vi "hw1-2.vi"() -> ()   [LabVIEW 2014]
panel:
  in  "Length of line 1":dbl
  in  "stop":bool
  out "2D Picture":picture
  in  "Angle 2":dbl(slide) scale=0.0..360.0
  in  "Length of line 2":dbl
  in  "Angle 1":dbl(slide) scale=0.0..360.0
  out "Line 1End y":dbl
  out "Line 1End x":dbl
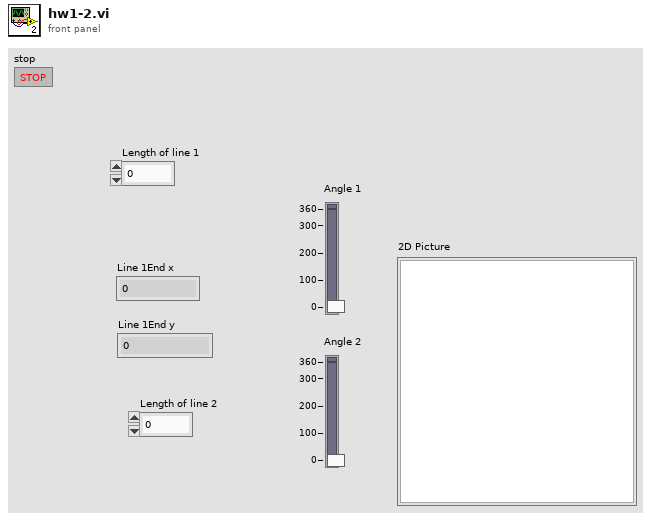
[diagram p1: front panel]
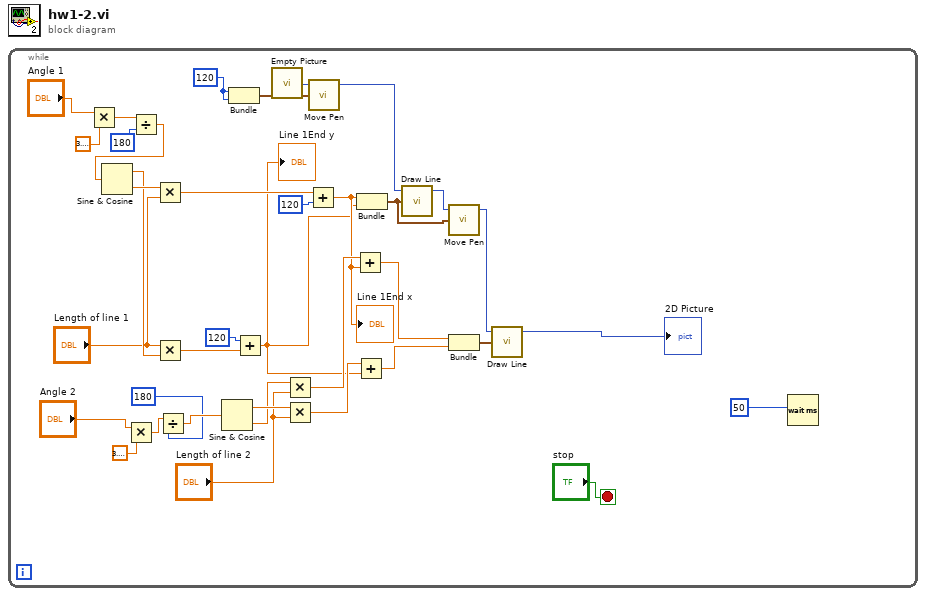
[diagram p0: block diagram]
diagram:
  n1 = while {
    stop <- "stop" stop-if-true
    w27 = 120
    n2 = Multiply(x="Angle 1", y=3.141592653589793) -> (x*y=w6:dbl)
    n3 = Multiply(x="Angle 2", y=3.141592653589793) -> (x*y=w2:dbl)
    n4 = Divide(x=w6, y=180) -> (x/y=w5:dbl)
    n5 = Sine & Cosine(0:w5) -> (1:w35:dbl, 2:w37:dbl)
    n6 = Multiply(x=w37, y="Length of line 1") -> (x*y=w36:dbl)
    n7 = Multiply(x="Length of line 1", y=w35) -> (x*y=w34:dbl)
    n8 = Divide(x=w2, y=180) -> (x/y=w3:dbl)
    n9 = Sine & Cosine(0:w3) -> (1:w33:dbl, 2:w32:dbl)
    n10 = Bundle(w27, w27) -> (w26:cluster{i32, i32})  [unwired: 1 in]
    n11 = Add(x=120, y=w34) -> (x+y=w14:dbl)
    "Line 1End y" <- w14
    n12 = call "Empty Picture"() -> ("empty picture"=w25:picture)
    n13 = Multiply(x=w32, y="Length of line 2") -> (x*y=w29:dbl)
    n14 = Multiply(x=w33, y="Length of line 2") -> (x*y=w30:dbl)
    n15 = Add(x=w36, y=120) -> (x+y=w20:dbl)
    "Line 1End x" <- w20
    n16 = call <vilib>:"Move Pen.vi"("new position"=w26, "picture"=w25) -> ("new picture"=w24:picture)  [unwired: 3 in]
    n17 = Add(x=w29, y=w20) -> (x+y=w13:dbl)
    n18 = Add(x=w30, y=w14) -> (x+y=w19:dbl)
    n19 = Bundle(w20, w14) -> (w12:cluster{dbl, dbl})  [unwired: 1 in]
    n20 = call <vilib>:"Draw Line.vi"("picture"=w24, "end point"=w12) -> ("new picture"=w23:picture)  [unwired: 7 in]
    n21 = call <vilib>:"Move Pen.vi"("new position"=w12, "picture"=w23) -> ("new picture"=w22:picture)  [unwired: 3 in]
    n22 = Bundle(w13, w19) -> (w18:cluster{dbl, dbl})  [unwired: 1 in]
    n23 = call <vilib>:"Draw Line.vi"("picture"=w22, "end point"=w18) -> ("new picture"=→"2D Picture":picture)  [unwired: 7 in]
    n24 = Wait (ms)(milliseconds to wait=50) -> ()  [unwired: 1 out]
  }
